vi "InstrumentSelection.vi"(8 "error in (no error)":errorcluster, 9 "Verify GPIB address":bool, 10 "Instrument type":T1(ring), 11 "Instrument name IN":string(combo)) -> (0 "error out":errorcluster, 1 "Instrument name OUT":string, 2 "LCR":refnum<class "LCRControl.lvclass">, 3 "Supply":refnum<class "SupplyControl.lvclass">, 4 "Switching":refnum<class "Switching.lvclass">, 5 "Multimeter":refnum<class "MultimeterControl.lvclass">)   [LabVIEW 2018, in "InstrControl.lvclass"]
uses:
  InstrControl.lvclass
  SupplyControl/SupplyControl.lvclass
  C:/Users/veral/Documents/itk-strip-sensor-qc/LabVIEW 2013/InstrControl/InstrControl.lvclass
  LCRControl/LCRControl.lvclass
  MultimeterControl/MultimeterControl.lvclass
  Switching/Switching.lvclass
  SupplyControl/Keithley 2410/KE2410.lvclass
  C:/Users/veral/Documents/itk-strip-sensor-qc/LabVIEW 2013/InstrControl/SupplyControl/SupplyControl.lvclass
  SupplyControl/Keithley 6517/KE6517.lvclass
  SupplyControl/Keithley 487/KE487.lvclass
  SupplyControl/Keithley 236 & 237/KE236.lvclass
  SupplyControl/Keithley237/KE237.lvclass
  LCRControl/WK6440B/WK6440B.lvclass
  C:/Users/veral/Documents/itk-strip-sensor-qc/LabVIEW 2013/InstrControl/LCRControl/LCRControl.lvclass
  LCRControl/WK6425/WK6425.lvclass
  LCRControl/HP4284A/HP4284A.lvclass
  MultimeterControl/Keithley 2000/KE2000.lvclass
  C:/Users/veral/Documents/itk-strip-sensor-qc/LabVIEW 2013/InstrControl/MultimeterControl/MultimeterControl.lvclass
  Switching/Pickering/Pickering.lvclass
  C:/Users/veral/Documents/itk-strip-sensor-qc/LabVIEW 2013/InstrControl/Switching/Switching.lvclass
  Switching/Keithley 3706A/KE3706A.lvclass
  InstrumentSetup.vi
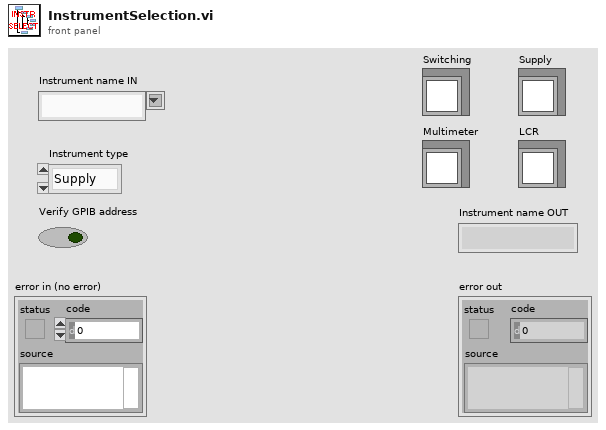
[diagram p1: front panel]
types:
  T1 = enum16{"Supply", "LCR", "Multimeter", "Switching"}
  T2 = cluster{"KE 2410":cluster{"Instrument name":string, "address":refnum<visa-resource-name>, "Instrument type":u16}, "KE 6517":cluster{"Instrument name":string, "address":refnum<visa-resource-name>, "Instrument type":u16}, "KE 487":cluster{"Instrument name":string, "address":refnum<visa-resource-name>, "Instrument type":u16}, "KE 236":cluster{"Instrument name":string, "address":refnum<visa-resource-name>, "Instrument type":u16}, "WK 6440B":cluster{"Instrument name":string, "address":refnum<visa-resource-name>, "Instrument type":u16}, "WK 6425":cluster{"Instrument name":string, "address":refnum<visa-resource-name>, "Instrument type":u16}, "Pickering Matrix":cluster{"Instrument name":string, "address":refnum<visa-resource-name>, "Instrument type":u16}, "KE 2000":cluster{"Instrument name":string, "address":refnum<visa-resource-name>, "Instrument type":u16}, "KE3706A Switching":cluster{"Instrument name":string, "address":refnum<visa-resource-name>, "Instrument type":u16}, "HP 4284A":cluster{"Instrument name":string, "address":refnum<visa-resource-name>, "Instrument type":u16}, "KE237":cluster{"Instrument name":string, "address":refnum<visa-resource-name>, "Instrument type":u16}}
  T3 = cluster{"Current Limit":sgl, "KE2410":refnum<class "KE2410.lvclass">}
  T4 = cluster{"Current Limit":u16, "KE6517":refnum<class "KE6517.lvclass">}
  T5 = cluster{"Compliance":u16, "Range:":u16, "KE487":refnum<class "KE487.lvclass">}
  T6 = cluster{"current \ncompliance level":dbl, "compliance/\nmeasurement range (auto:0)":u16, "KE236":refnum<class "KE236.lvclass">}
  T7 = cluster{"current \ncompliance level":dbl, "compliance/\nmeasurement range (auto:0)":u16, "KE237":refnum<class "KE237.lvclass">}
  T8 = cluster{"RC Configuration":u16, "AC amplitude [V]":dbl, "AC frequency [Hz]":i32, "WK6440B":refnum<class "WK6440B.lvclass">}
  T9 = cluster{"RC Configuration":u16, "AC amplitude [V]":dbl, "AC frequency [Hz]":i32, "WK6425":refnum<class "WK6425.lvclass">}
  T10 = cluster{"RC Configuration":u16, "AC amplitude [V]":dbl, "Consider OC":bool, "Consider SC":bool, "AC frequency [Hz]":i32, "HP4284A":refnum<class "HP4284A.lvclass">}
  T11 = cluster{"Range":u16, "Range Value":dbl, "Function":u16, "KE2000":refnum<class "KE2000.lvclass">}
  T12 = cluster{"Matrix address":string, "Mux1 address":string, "Mux2 address":string, "Pickering":refnum<class "Pickering.lvclass">, "Matrix X Channels":cluster{"Bias Supply / SMU LO":i32, "Bias Supply / SMU HI":i32, "CV Box LO":i32, "CV Box HI":i32, "CV Box LO IN":i32, "CV Box HI IN":i32, "Volt meter LO":i32, "Volt meter HI":i32, "Mux1 C1":i32, "Mux1 C2":i32, "Mux2 C1":i32, "Mux2 C2":i32}}
  T13 = cluster{"Mux1 slot":string, "Mux2 slot":string, "KE3706A":refnum<class "KE3706A.lvclass">}
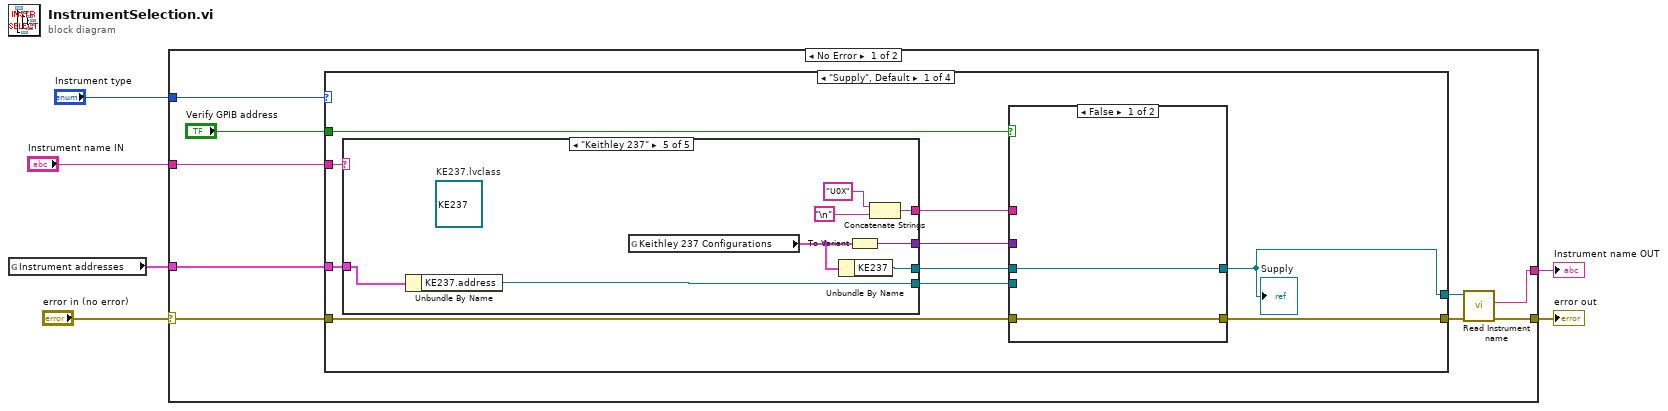
[diagram p0: block diagram]
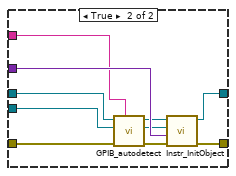
[diagram p2: hidden frame]
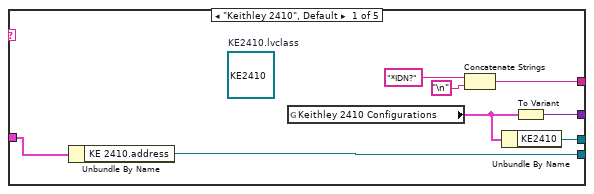
[diagram p3: hidden frame]
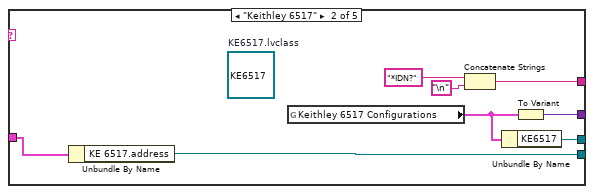
[diagram p4: hidden frame]
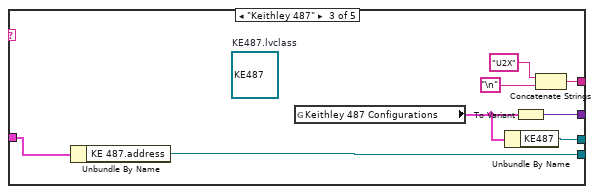
[diagram p5: hidden frame]
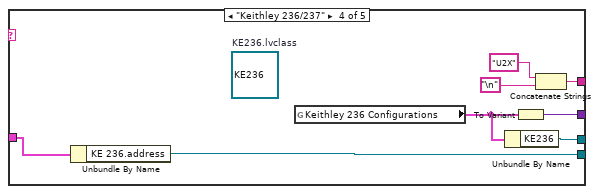
[diagram p6: hidden frame]
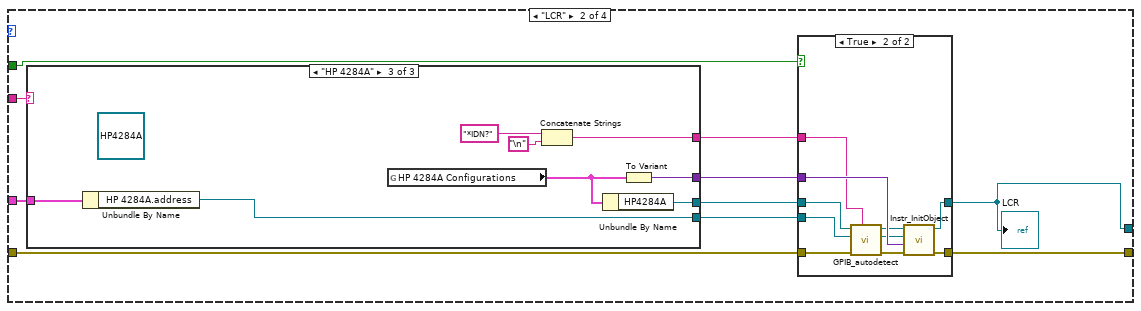
[diagram p7: hidden frame]
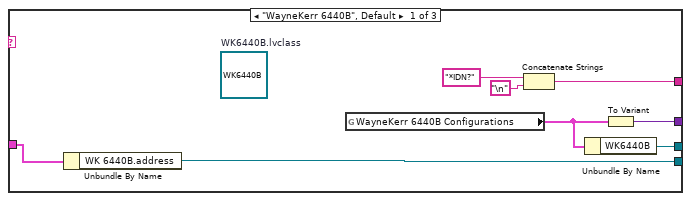
[diagram p9: hidden frame]
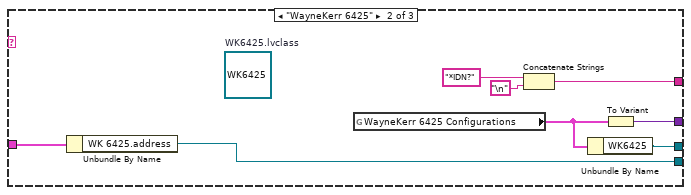
[diagram p10: hidden frame]
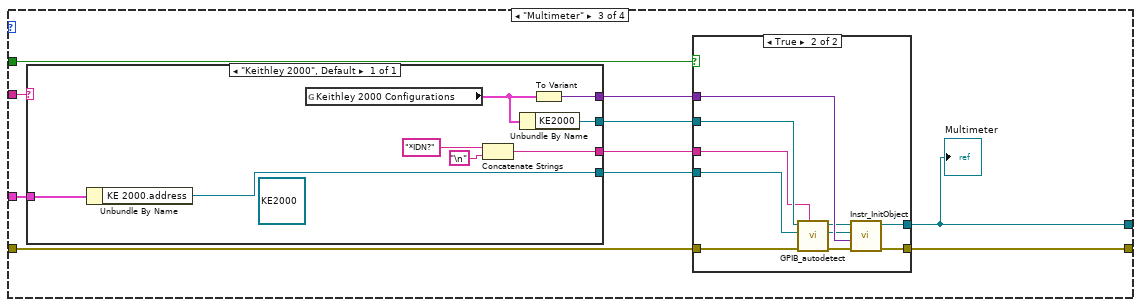
[diagram p11: hidden frame]
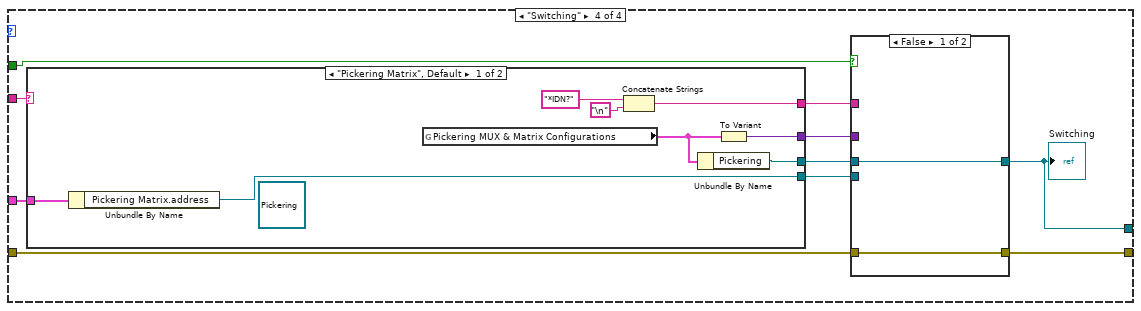
[diagram p13: hidden frame]
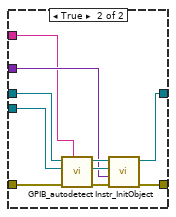
[diagram p14: hidden frame]
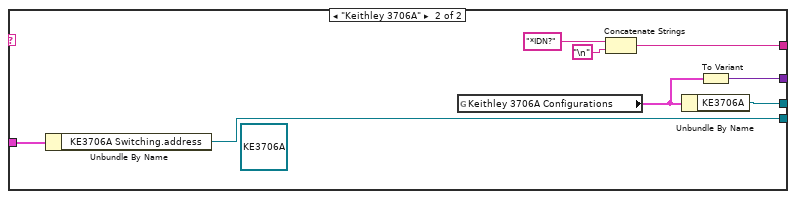
[diagram p15: hidden frame]
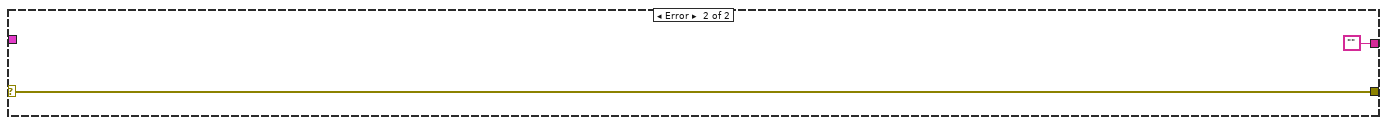
[diagram p16: hidden frame]
diagram:
  n1 = global read "InstrumentSetup.vi" "Instrument addresses"() -> (w1:T2)
  n2 = case shown="No Error" "error in (no error)" {
    selector: "error in (no error)" -> [w13 w193]
    tunnel: [w14 w193] -> w5
    tunnel: [w15 ""] -> w4
    tunnel: "Instrument type" -> [w10 _]
    tunnel: "Instrument name IN" -> [w9 _]
    tunnel: w1 -> [w8 _]
    frame No Error {
      n3 = case shown="\"Supply\", Default" w10 {
        tunnel: w9 -> [w25 w87 w133 w158]
        tunnel: [w24 w85 w131 w162] -> w12
        tunnel: w13 -> [w18 w82 w126 w159]
        tunnel: [w23 w86 w132 w163] -> w11
        tunnel: w8 -> [w22 w84 w130 w161]
        tunnel: "Verify GPIB address" -> [w16 w78 w124 w154]
        frame "Supply", Default {
          n4 = case shown="\"Keithley 237\"" w25 {
            tunnel: [w42 w49 w57 w65 w73] -> w19
            tunnel: w22 -> [w45 w53 w61 w69 w77]
            tunnel: [w44 w52 w60 w68 w76] -> w20
            tunnel: [w43 w51 w59 w67 w75] -> w21
            tunnel: [w38 w46 w54 w62 w70] -> w17
            frame "Keithley 2410", Default {
              (unwired) refnum<class "KE2410.lvclass"> refnum  # KE2410.lvclass
              n5 = Unbundle By Name(w45) -> ("KE 2410.address"=w44:refnum<visa-resource-name>)
              n6 = global read "InstrumentSetup.vi" "Keithley 2410 Configurations"() -> (w41:T3)
              n7 = Concatenate Strings("*IDN?" ("regular expression"), "\n") -> (w38:string)
              n8 = Unbundle By Name(w41) -> ("KE2410"=w42:refnum<class "KE2410.lvclass">)
              n9 = To Variant(anything=w41) -> (Variant=w43:variant)
            }
            frame "Keithley 6517" {
              (unwired) refnum<class "KE6517.lvclass"> refnum  # KE6517.lvclass
              n10 = Unbundle By Name(w53) -> ("KE 6517.address"=w52:refnum<visa-resource-name>)
              n11 = global read "InstrumentSetup.vi" "Keithley 6517 Configurations"() -> (w50:T4)
              n12 = Concatenate Strings("*IDN?" ("regular expression"), "\n") -> (w46:string)
              n13 = Unbundle By Name(w50) -> ("KE6517"=w49:refnum<class "KE6517.lvclass">)
              n14 = To Variant(anything=w50) -> (Variant=w51:variant)
            }
            frame "Keithley 487" {
              (unwired) refnum<class "KE487.lvclass"> refnum  # KE487.lvclass
              n15 = Unbundle By Name(w61) -> ("KE 487.address"=w60:refnum<visa-resource-name>)
              n16 = global read "InstrumentSetup.vi" "Keithley 487 Configurations"() -> (w58:T5)
              n17 = Unbundle By Name(w58) -> ("KE487"=w57:refnum<class "KE487.lvclass">)
              n18 = To Variant(anything=w58) -> (Variant=w59:variant)
              n19 = Concatenate Strings("U2X" ("regular expression"), "\n") -> (w54:string)
            }
            frame "Keithley 236/237" {
              (unwired) refnum<class "KE236.lvclass"> refnum  # KE236.lvclass
              n20 = Unbundle By Name(w69) -> ("KE 236.address"=w68:refnum<visa-resource-name>)
              n21 = global read "InstrumentSetup.vi" "Keithley 236 Configurations"() -> (w66:T6)
              n22 = Unbundle By Name(w66) -> ("KE236"=w65:refnum<class "KE236.lvclass">)
              n23 = To Variant(anything=w66) -> (Variant=w67:variant)
              n24 = Concatenate Strings("U2X" ("regular expression"), "\n") -> (w62:string)
            }
            frame "Keithley 237" {
              (unwired) refnum<class "KE237.lvclass"> refnum  # KE237.lvclass
              n25 = Unbundle By Name(w77) -> ("KE237.address"=w76:refnum<visa-resource-name>)
              n26 = global read "InstrumentSetup.vi" "Keithley 237 Configurations"() -> (w74:T7)
              n27 = Unbundle By Name(w74) -> ("KE237"=w73:refnum<class "KE237.lvclass">)
              n28 = To Variant(anything=w74) -> (Variant=w75:variant)
              n29 = Concatenate Strings("U0X" ("regular expression"), "\n") -> (w70:string)
            }
          }
          n30 = case shown="False" w16 {
            tunnel: [w27 w37] -> w24
            tunnel: [w26 w36] -> w23
            tunnel: w21 -> [_ w35]
            tunnel: w20 -> [_ w34]
            tunnel: w19 -> [w27 w32]
            tunnel: w18 -> [w26 w30]
            tunnel: w17 -> [_ w28]
            frame False {
            }
            frame True {
              n31 = call-dynamic "GPIB_autodetect.vi"("ID command"=w28, "error in (no error)"=w30, "Instrument address in"=w34, "InstrControl in"=w32) -> ("error out"=w29:errorcluster, "Instrument address out"=w33:refnum<visa-resource-name>, "InstrControl out"=w31:refnum<class "SupplyControl.lvclass">)  [unwired: 5 in]
              n32 = call-dynamic "Instr_InitObject.vi"("error in (no error)"=w29, "Instrument Configuration"=w35, "Instrument address"=w33, "SupplyControl in"=w31) -> ("error out"=w36:errorcluster, "SupplyControl out"=w37:refnum<class "SupplyControl.lvclass">)  [unwired: 6 in]
            }
          }
          "Supply" <- w24
        }
        frame "LCR" {
          n33 = case shown="\"HP 4284A\"" w87 {
            tunnel: [w103 w111 w119] -> w80
            tunnel: w84 -> [w107 w115 w123]
            tunnel: [w106 w114 w122] -> w81
            tunnel: [w105 w113 w121] -> w83
            tunnel: [w100 w108 w116] -> w79
            frame "WayneKerr 6440B", Default {
              (unwired) refnum<class "WK6440B.lvclass"> refnum  # WK6440B.lvclass
              n34 = Unbundle By Name(w107) -> ("WK 6440B.address"=w106:refnum<visa-resource-name>)
              n35 = global read "InstrumentSetup.vi" "WayneKerr 6440B Configurations"() -> (w104:T8)
              n36 = Concatenate Strings("*IDN?" ("regular expression"), "\n") -> (w100:string)
              n37 = Unbundle By Name(w104) -> ("WK6440B"=w103:refnum<class "WK6440B.lvclass">)
              n38 = To Variant(anything=w104) -> (Variant=w105:variant)
            }
            frame "WayneKerr 6425" {
              (unwired) refnum<class "WK6425.lvclass"> refnum  # WK6425.lvclass
              n39 = Unbundle By Name(w115) -> ("WK 6425.address"=w114:refnum<visa-resource-name>)
              n40 = global read "InstrumentSetup.vi" "WayneKerr 6425 Configurations"() -> (w112:T9)
              n41 = Concatenate Strings("*IDN?" ("regular expression"), "\n") -> (w108:string)
              n42 = Unbundle By Name(w112) -> ("WK6425"=w111:refnum<class "WK6425.lvclass">)
              n43 = To Variant(anything=w112) -> (Variant=w113:variant)
            }
            frame "HP 4284A" {
              (unwired) refnum<class "HP4284A.lvclass"> refnum ("HP4284A.lvclass")
              n44 = Unbundle By Name(w123) -> ("HP 4284A.address"=w122:refnum<visa-resource-name>)
              n45 = global read "InstrumentSetup.vi" "HP 4284A Configurations"() -> (w120:T10)
              n46 = Concatenate Strings("*IDN?" ("regular expression"), "\n") -> (w116:string)
              n47 = Unbundle By Name(w120) -> ("HP4284A"=w119:refnum<class "HP4284A.lvclass">)
              n48 = To Variant(anything=w120) -> (Variant=w121:variant)
            }
          }
          n49 = case shown="True" w78 {
            tunnel: [w88 w99] -> w86
            tunnel: [w89 w98] -> w85
            tunnel: w83 -> [_ w97]
            tunnel: w82 -> [w88 w96]
            tunnel: w81 -> [_ w94]
            tunnel: w80 -> [w89 w92]
            tunnel: w79 -> [_ w90]
            frame False {
            }
            frame True {
              n50 = call-dynamic "GPIB_autodetect.vi"("ID command"=w90, "error in (no error)"=w96, "Instrument address in"=w94, "InstrControl in"=w92) -> ("error out"=w95:errorcluster, "Instrument address out"=w93:refnum<visa-resource-name>, "InstrControl out"=w91:refnum<class "LCRControl.lvclass">)  [unwired: 5 in]
              n51 = call-dynamic "Instr_InitObject.vi"("error in (no error)"=w95, "Instrument Configuration"=w97, "Instrument address"=w93, "LCRControl in"=w91) -> ("error out"=w99:errorcluster, "LCRControl out"=w98:refnum<class "LCRControl.lvclass">)  [unwired: 6 in]
            }
          }
          "LCR" <- w85
        }
        frame "Multimeter" {
          n52 = case shown="\"Keithley 2000\", Default" w133 {
            tunnel: [w149] -> w127
            tunnel: w130 -> [w153]
            tunnel: [w152] -> w128
            tunnel: [w151] -> w129
            tunnel: [w146] -> w125
            frame "Keithley 2000", Default {
              (unwired) refnum<class "KE2000.lvclass"> refnum ("KE2000.lvclass")
              n53 = Unbundle By Name(w153) -> ("KE 2000.address"=w152:refnum<visa-resource-name>)
              n54 = global read "InstrumentSetup.vi" "Keithley 2000 Configurations"() -> (w150:T11)
              n55 = Concatenate Strings("*IDN?" ("regular expression"), "\n") -> (w146:string)
              n56 = Unbundle By Name(w150) -> ("KE2000"=w149:refnum<class "KE2000.lvclass">)
              n57 = To Variant(anything=w150) -> (Variant=w151:variant)
            }
          }
          n58 = case shown="True" w124 {
            tunnel: [w135 w145] -> w132
            tunnel: [w134 w144] -> w131
            tunnel: w129 -> [_ w143]
            tunnel: w128 -> [_ w142]
            tunnel: w127 -> [w134 w139]
            tunnel: w126 -> [w135 w138]
            tunnel: w125 -> [_ w136]
            frame False {
            }
            frame True {
              n59 = call-dynamic "GPIB_autodetect.vi"("ID command"=w136, "error in (no error)"=w138, "Instrument address in"=w142, "InstrControl in"=w139) -> ("error out"=w137:errorcluster, "Instrument address out"=w141:refnum<visa-resource-name>, "InstrControl out"=w140:refnum<class "KE2000.lvclass">)  [unwired: 5 in]
              n60 = call-dynamic "Instr_InitObject.vi"("error in (no error)"=w137, "Instrument Configuration"=w143, "Instrument address"=w141, "KE2000 in"=w140) -> ("error out"=w145:errorcluster, "KE2000 out"=w144:refnum<class "KE2000.lvclass">)  [unwired: 6 in]
            }
          }
          "Multimeter" <- w131
        }
        frame "Switching" {
          n61 = case shown="\"Pickering Matrix\", Default" w158 {
            tunnel: w161 -> [w183 w188]
            tunnel: [w182 w187] -> w160
            tunnel: [w180 w185] -> w157
            tunnel: [w179 w189] -> w156
            tunnel: [w176 w186] -> w155
            frame "Pickering Matrix", Default {
              (unwired) refnum<class "Pickering.lvclass"> refnum ("Pickering")
              n62 = Unbundle By Name(w183) -> ("Pickering Matrix.address"=w182:refnum<visa-resource-name>)
              n63 = global read "InstrumentSetup.vi" "Pickering MUX & Matrix Configurations"() -> (w181:T12)
              n64 = Concatenate Strings("*IDN?" ("regular expression"), "\n") -> (w176:string)
              n65 = Unbundle By Name(w181) -> ("Pickering"=w179:refnum<class "Pickering.lvclass">)
              n66 = To Variant(anything=w181) -> (Variant=w180:variant)
            }
            frame "Keithley 3706A" {
              (unwired) refnum<class "KE3706A.lvclass"> refnum ("KE3700A in")
              n67 = Unbundle By Name(w188) -> ("KE3706A Switching.address"=w187:refnum<visa-resource-name>)
              n68 = global read "InstrumentSetup.vi" "Keithley 3706A Configurations"() -> (w191:T13)
              n69 = Concatenate Strings("*IDN?" ("regular expression"), "\n") -> (w186:string)
              n70 = Unbundle By Name(w191) -> ("KE3706A"=w189:refnum<class "KE3706A.lvclass">)
              n71 = To Variant(anything=w191) -> (Variant=w185:variant)
            }
          }
          n72 = case shown="False" w154 {
            tunnel: [w165 w175] -> w163
            tunnel: [w164 w174] -> w162
            tunnel: w160 -> [_ w172]
            tunnel: w159 -> [w165 w169]
            tunnel: w157 -> [_ w168]
            tunnel: w156 -> [w164 w167]
            tunnel: w155 -> [_ w166]
            frame False {
            }
            frame True {
              n73 = call-dynamic "GPIB_autodetect.vi"("ID command"=w166, "error in (no error)"=w169, "Instrument address in"=w172, "InstrControl in"=w167) -> ("error out"=w171:errorcluster, "Instrument address out"=w170:refnum<visa-resource-name>, "InstrControl out"=w173:refnum<class "Switching.lvclass">)  [unwired: 5 in]
              n74 = call-dynamic "Instr_InitObject.vi"("error in (no error)"=w171, "Instrument Configuration"=w168, "Instrument address"=w170, "Switching in"=w173) -> ("error out"=w175:errorcluster, "Switching out"=w174:refnum<class "Switching.lvclass">)  [unwired: 6 in]
            }
          }
          "Switching" <- w162
        }
      }
      n75 = call-dynamic "Read Instrument name.vi"("error in (no error)"=w11, "InstControl in"=w12) -> ("error out"=w14:errorcluster, "Instrument name"=w15:string)  [unwired: 7 in, 1 out]
    }
    frame Error {
    }
  }
  "error out" <- w5
  "Instrument name OUT" <- w4
